vi "PerformCalibrationMultiMixture.vi"(0 "MFCS_EZ":T3, 1 "Total Flow Setpoint":dbl, 2 "Ctr Water Valve":u16(ring) items=["A1", "A2", "A3", "A4", "B1", "B2", "B3", "B4", "B5", "B6", "B7", "B8", "A5", "A6", "A7", "A8"], 3 "Calibration Mode":T2(ring), 5 "Calibration Refs":T1, 7 "Manual Default Set Pressures":dbl[](array[numeric]), 12 "Total Odor Flow":dbl, 13 "Water Mix Valve":u16(ring) items=["A1", "A2", "A3", "A4", "B1", "B2", "B3", "B4", "B5", "B6", "B7", "B8", "A5", "A6", "A7", "A8", ""]) -> (4 "Ctr Pressure":dbl, 6 "Set Pressures Out":dbl[](array[numeric]), 10 "New Manual Pressure":dbl[](array[numeric]), 15 "Aborted?":bool)   [LabVIEW 2016]
uses:
  <userlib>/Fluigent/Fluigent MFCS/FluigentMFCS_Full.llb/_EZmfcsRefNum.ctl
  <userlib>/Fluigent/Fluigent MFCS/FluigentMFCS_Full.llb/_EZmfcsEnum.ctl
  <userlib>/Fluigent/Fluigent MFCS/FluigentMFCS_Full.llb/MFCS_EZ Write Channel Pressure.vi
  <userlib>/Fluigent/Fluigent MFCS/FluigentMFCS_Full.llb/MFCS_EZ Read All Channels Pressure.vi
  <vilib>/Utility/miscctls.llb/LVStringsAndValuesArrayTypeDef.ctl
panel:
  out "odor starting pressure":dbl
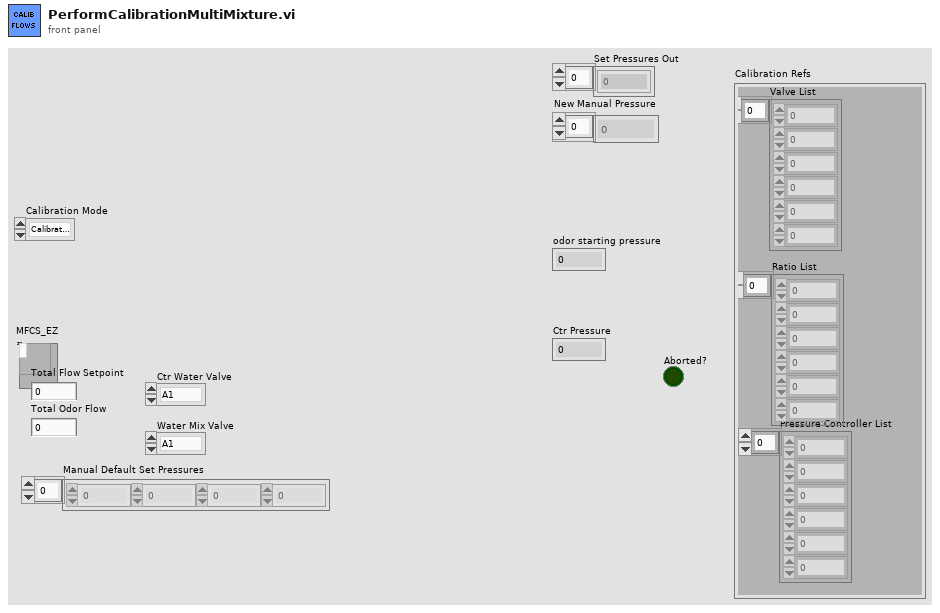
[diagram p1: front panel]
types:
  T1 = cluster{"Pressure Controller List":u8[], "Ratio List":dbl[], "Valve List":u16[]}
  T2 = enum16{"Calibrate All", "Control Only", "Odors Only"}
  T3 = typedef "_EZmfcsRefNum.ctl" = refnum<k1>
  T4 = cluster{enum16{"A", "B", "C"}[], enum16{"1", "2", "3", "4", "5", "6", "7", "8"}[], bool[]}[]
  T5 = typedef "LVStringsAndValuesArrayTypeDef.ctl" = cluster{"String":string, "Value":ext}[]
  T6 = enum16{"Release", "Create", "Send", "Wait", "Cancel"}
  T7 = cluster{enum16{"A", "B", "C"}[], enum16{"1", "2", "3", "4", "5", "6", "7", "8"}[], bool[]}
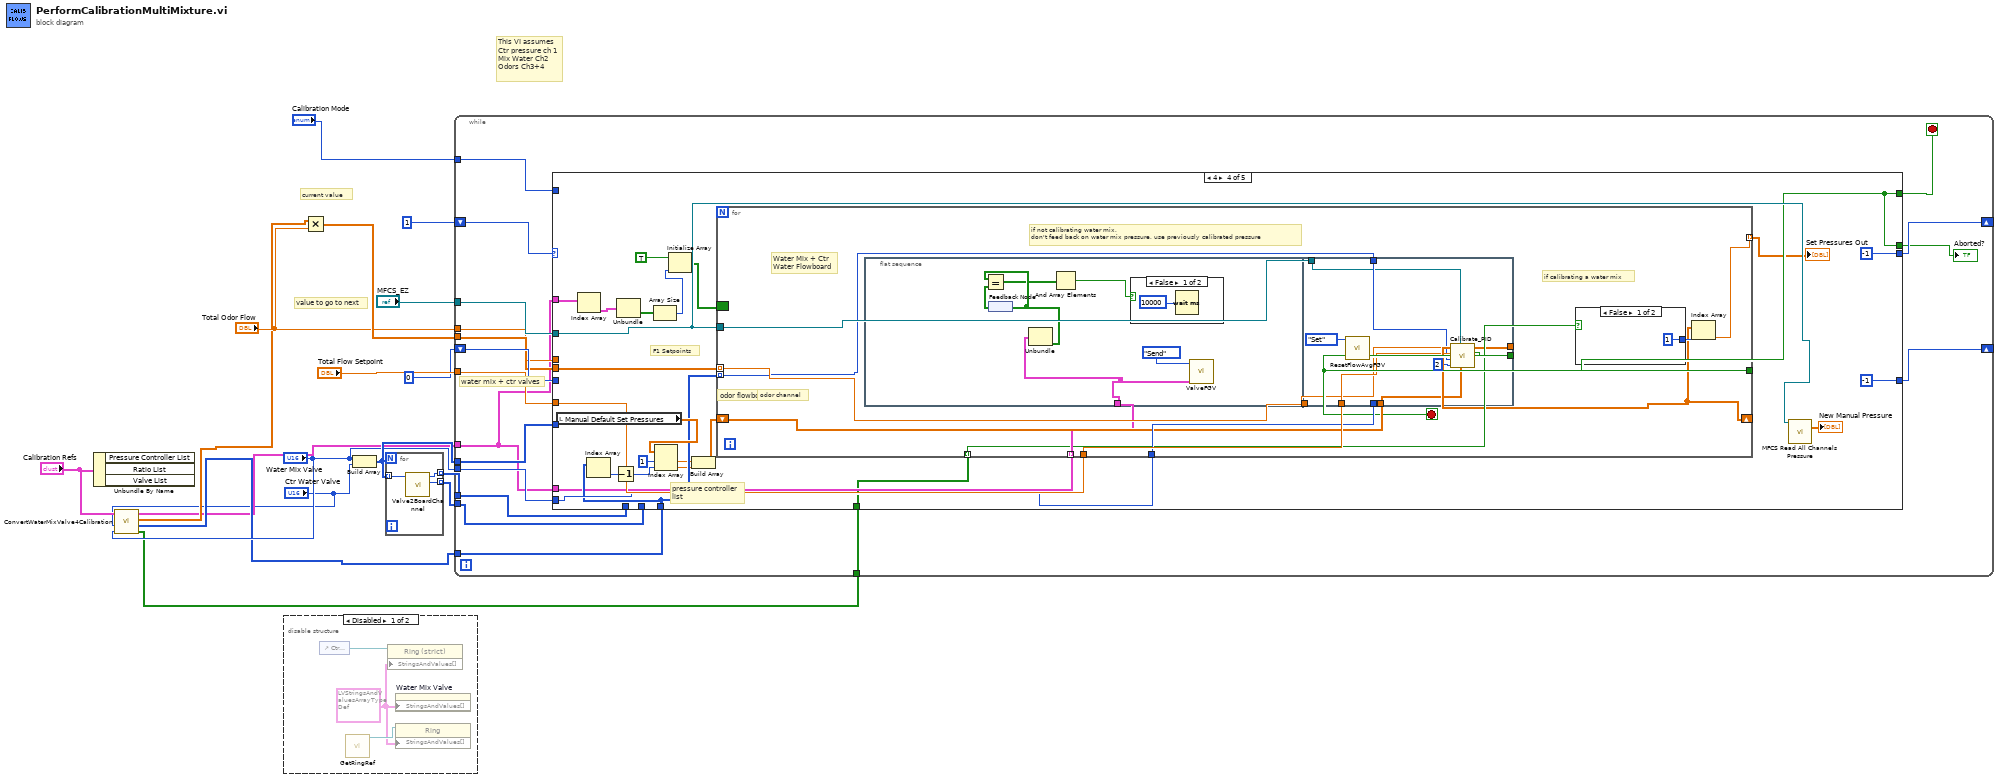
[diagram p0: block diagram]
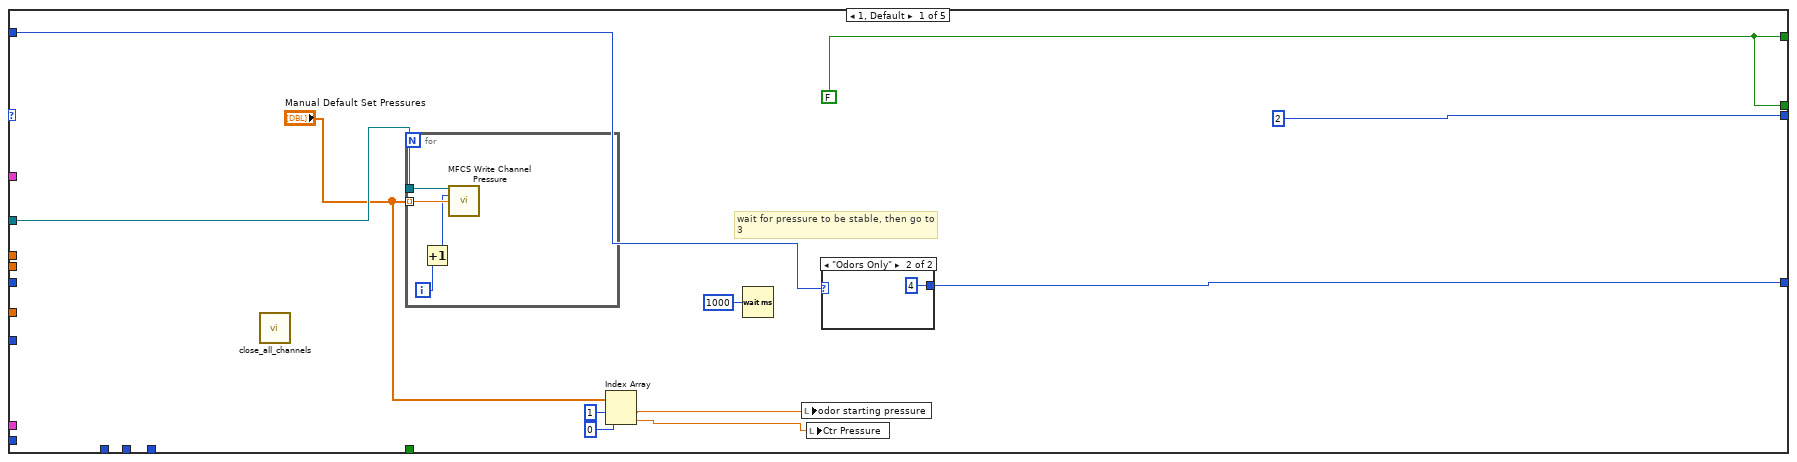
[diagram p3: hidden frame]
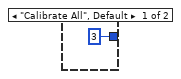
[diagram p4: hidden frame]
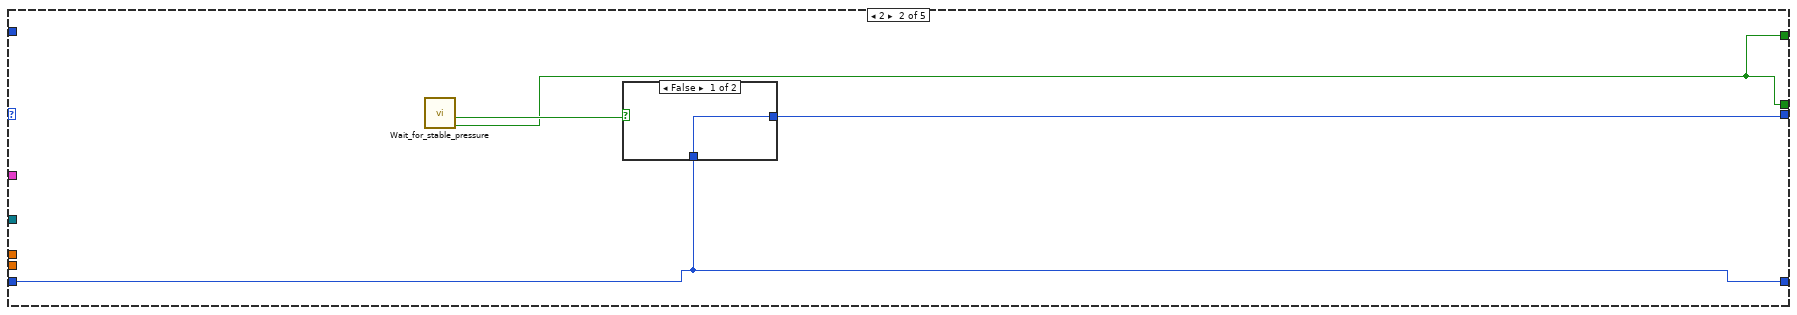
[diagram p5: hidden frame]
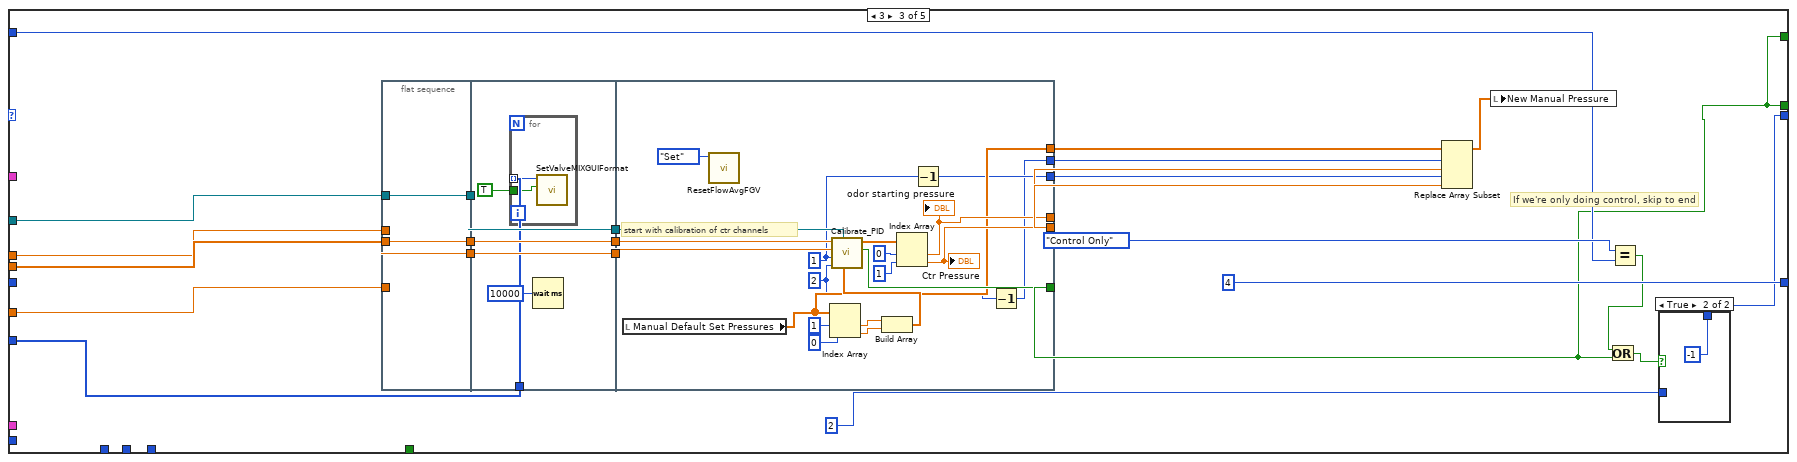
[diagram p7: hidden frame]
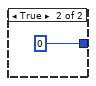
[diagram p9: hidden frame]
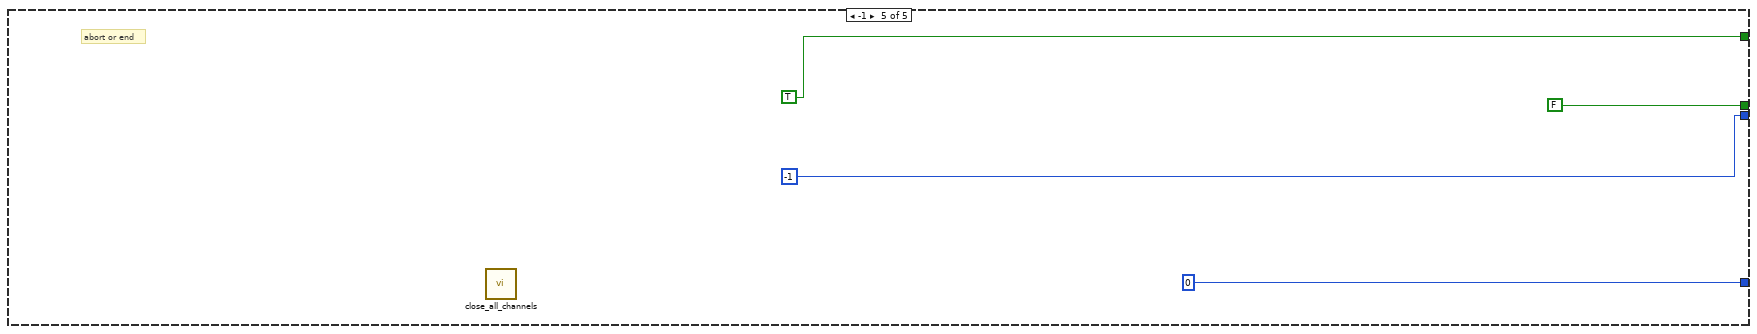
[diagram p11: hidden frame]
diagram:
  # "This VI assumes \nCtr pressure ch 1\nMix Water Ch2\nOdors Ch3+4"
  # "current value"
  # "value to go to next"
  n1 = Unbundle By Name("Calibration Refs") -> ()  [unwired: 3 out]
  n2 = call "ConvertWaterMixValve4Calibration.vi"("Water Mix Valve"="Water Mix Valve", "Ctr Water Valve"="Ctr Water Valve", "Calibration Refs"="Calibration Refs") -> ("Water Calibration?"=w2:bool[], "PressList"=w5:u8[], "RatioList"=w4:dbl[], "Valve Signal Array"=w3:T4)  [unwired: 5 in]
  n3 = disable-structure shown="Disabled" {
    frame Disabled {
      w18 = T5 [{"String"="A1", "Value"=0.0}, {"String"="A2", "Value"=1.0}, {"String"="A3", "Value"=2.0}, {"String"="A4", "Value"=3.0}, {"String"="B1", "Value"=4.0}, {"String"="B2", "Value"=5.0}, {"String"="B3", "Value"=6.0}, {"String"="B4", "Value"=7.0}, {"String"="B5", "Value"=8.0}, {"String"="B6", "Value"=9.0}, {"String"="B7", "Value"=10.0}, {"String"="B8", "Value"=11.0}, {"String"="A5", "Value"=12.0}] ("Master Valves")
      n4 = control-ref of="Ctr Water Valve"() -> (w19:refnum<vi>)
      n5 = call "GetRingRef.vi"() -> ("Ring Reference"=w20:refnum<vi>, "Array Reference"=w21:refnum<vi>)  [unwired: 9 in, 1 out]
      n6 = property on="Property Node" class="Ring (strict)"(reference=w19, "StringsAndValues[]"=w18) -> ()  [unwired: 1 in, 2 out]
      n7 = property on="Water Mix Valve" class="Ring (strict)"("StringsAndValues[]"=w18) -> ()  [unwired: 2 in, 2 out]
      n8 = property class="Ring"(reference=w20, "StringsAndValues[]"=w18) -> ()  [unwired: 1 in, 2 out]
    }
    frame Enabled {
    }
  }
  n9 = Multiply(x=w4, y="Total Odor Flow") -> (x*y=w10:dbl[])
  n10 = Build Array("Water Mix Valve", "Ctr Water Valve") -> (w13:u16[])
  n11 = for {
    tunnel: w13 -> [w24] mode=indexing
    tunnel: [w23] -> w12 mode=indexing
    tunnel: [w22] -> w11 mode=indexing
    n12 = call "Valve2BoardChannel.vi"("ValveID"=w24) -> ("Channel"=w22:enum16{"1", "2", "3", "4", "5", "6", "7", "8"}, "Flowboard"=w23:enum16{"A", "B", "C"})  [unwired: 9 in]
  }
  n13 = while {
    tunnel: "MFCS_EZ" -> [w42]
    tunnel: "Total Flow Setpoint" -> [w41]
    shift-right: [w39] -> _
    shift-left: 1 -> [w40]
    tunnel: w13 -> [w38]
    shift-right: [w37] -> _
    shift-left: 0 -> [w36]
    tunnel: w5 -> [w29]
    tunnel: w12 -> [w35]
    tunnel: w11 -> [w34]
    tunnel: w10 -> [w33]
    tunnel: "Water Mix Valve" -> [w31]
    tunnel: "Total Odor Flow" -> [w32]
    tunnel: "Calibration Mode" -> [w30]
    tunnel: w3 -> [w25]
    tunnel: w2 -> [w28]
    stop <- w27 stop-if-true
    # "pressure controller \nlist"
    # "water mix + ctr valves"
    n14 = case shown="4" w40 {
      tunnel: w42 -> [w52 _ w90 w133 _]
      tunnel: w33 -> [_ _ w89 w147 _]
      tunnel: w41 -> [_ _ w88 w148 _]
      tunnel: [w43 w60 w66 w131 TRUE] -> w27
      tunnel: [2 w63 w78 -1 -1] -> w39
      tunnel: w38 -> [_ _ w73 _ _]
      tunnel: [w51 w62 4 -1 0] -> w37
      tunnel: w36 -> [_ w62 _ _ _]
      tunnel: w29 -> [_ _ _ w140 _]
      tunnel: w35 -> [_ _ _ _ _]
      tunnel: w34 -> [_ _ _ _ _]
      tunnel: w31 -> [_ _ _ w146 _]
      tunnel: w32 -> [_ _ w81 _ _]
      tunnel: w30 -> [w49 _ w75 _ _]
      tunnel: w25 -> [_ _ _ w135 _]
      tunnel: w28 -> [_ _ _ w134 _]
      tunnel: [w43 w60 w66 w131 FALSE ("Aborted?")] -> w26
      tunnel: w25 -> [_ _ _ w129 _]
      frame 1, Default {
        w43 = FALSE
        # "wait for pressure to be stable, then go to\n3"
        n15 = call "close_all_channels.vi"() -> ()  [unwired: 12 in]
        n16 = for {
          tunnel: "Manual Default Set Pressures" -> [w59] mode=indexing
          tunnel: w52 -> [w57]
          i -> [w58]
          n17 = Increment(x=w58) -> (x+1=w56:i32)
          n18 = call-poly <userlib>:"MFCS Write Channel Pressure.vi"("MFCS_EZ"=w57, "Channel Number (default=1)"=w56, "Pressure (mBar)"=w59) -> ()  [unwired: 11 in, 2 out]
        }
        n19 = Index Array(array="Manual Default Set Pressures", index #1=1 ("index"), index #2=0 ("index")) -> (element #1=w46:dbl, element #2=w45:dbl)
        n20 = Wait (ms)(milliseconds to wait=u32 1000) -> ()  [unwired: 1 out]
        n21 = local write "odor starting pressure"(w46) -> ()
        n22 = local write "Ctr Pressure"(w45) -> ()
        n23 = case shown="\"Odors Only\"" w49 {
          tunnel: [3 4] -> w51
          frame "Calibrate All", Default {
          }
          frame "Odors Only" {
          }
        }
      }
      frame 2 {
        n24 = call "Wait_for_stable_pressure.vi"() -> ("Aborted?"=w60:bool, "Pressure Stable?"=w61:bool)  [unwired: 8 in]
        n25 = case shown="False" w61 {
          tunnel: [w64 w65] -> w63
          tunnel: w62 -> [w64 w65]
          frame False {
          }
          frame True {
          }
        }
      }
      frame 3 {
        # "If we're only doing control, skip to end"
        n26 = flat-sequence {
          tunnel: w88 -> [w94]
          tunnel: w89 -> [_]
          tunnel: w90 -> [w95]
          tunnel: [w95] -> w87
          tunnel: [w94] -> w84
          tunnel: w81 -> [w93]
          tunnel: [w93] -> w80
          tunnel: w87 -> [w101]
          tunnel: [w101] -> w86
          tunnel: [w100] -> w85
          tunnel: w84 -> [w99]
          tunnel: [w99] -> w83
          tunnel: w73 -> [w97]
          tunnel: w80 -> [w100]
          tunnel: w86 -> [w123]
          tunnel: w85 -> [w122]
          tunnel: w83 -> [w121]
          tunnel: [w114] -> w66
          tunnel: [w104] -> w72
          tunnel: [w105] -> w71
          tunnel: [w110] -> w70
          tunnel: [w109] -> w69
          tunnel: [w108] -> w67
          frame #0 {
          }
          frame #1 {
            n27 = for {
              tunnel: TRUE ("State") -> [w103]
              tunnel: w97 -> [w102] mode=indexing
              n28 = call "SetValveMIXGUIFormat.vi"("State"=w103, "ValveID"=w102) -> ()  [unwired: 10 in]
            }
            n29 = Wait (ms)(milliseconds to wait=u32 10000) -> ()  [unwired: 1 out]
          }
          frame #2 {
            w106 = i16 1 ("Odor Mix Pressure Channel")
            w107 = i16 2 ("Water Mix Pressure Channel")
            # "start with calibration of ctr channels"
            n30 = local read "Manual Default Set Pressures"() -> (w108:dbl[])
            n31 = call "ResetFlowAvgFGV.vi"("Action"=enum16{"Create", "Set", "Wait"}."Set") -> ()  [unwired: 10 in, 1 out]
            n32 = Index Array(array=w108, index #1=1 ("index"), index #2=0 ("index")) -> (element #1=w116:dbl, element #2=w117:dbl)
            n33 = Build Array(w116, w117) -> (w115:dbl[])
            n34 = call "Calibrate_PID.vi"("Starting Pressure"=w115, "MFCS_EZ"=w123, "Water Mix Pressure Channel"=w107, "Odor Mix Pressure Channel"=w106, "Ftot Setpoint"=w121, "F1 Setpoint"=w122) -> ("Aborted?"=w114:bool, "Set Pressure Out"=w120:dbl[])  [unwired: 4 in]
            n35 = Index Array(array=w120, index #1=0 ("index"), index #2=1 ("index")) -> (element #1=w109:dbl, element #2=w110:dbl)
            "Ctr Pressure" <- w110
            "odor starting pressure" <- w109
            n36 = Decrement(x=w106) -> (x-1=w105:i16)
            n37 = Decrement(x=w107) -> (x-1=w104:i16)
          }
        }
        n38 = Replace Array Subset(array=w67, new element #1=w69, index #1=w72, new element #2=w70, index #2=w71) -> (w68:dbl[])
        n39 = local write "New Manual Pressure"(w68) -> ()
        n40 = Equal?(x=T2."Control Only" ("Calibration Mode"), y=w75) -> (x = y?=w74:bool)
        n41 = Or(x=w74, y=w66) -> (x .or. y?=w77:bool)
        n42 = case shown="True" w77 {
          tunnel: 2 -> [w91 _]
          tunnel: [w91 -1] -> w78
          frame False {
          }
          frame True {
          }
        }
      }
      frame 4 {
        # "F1 Setpoints"
        n43 = local read "Manual Default Set Pressures"() -> (w142:dbl[])
        n44 = Index Array(array=w129) -> (element=w128:T7)  [unwired: 1 in]
        n45 = Index Array(array=w140) -> (element=w139:u8)  [unwired: 1 in]
        n46 = Decrement(x=w139) -> (x-1=w138:u8)
        n47 = Unbundle(w128) -> (w127:bool[])  [unwired: 2 out]
        n48 = Array Size(array=w127) -> (size(s)=w126:i32)
        n49 = Index Array(array=w142, index #1=1 ("index"), index #2=w138) -> (element #1=w136:dbl, element #2=w137:dbl)
        n50 = Initialize Array(TRUE, w126) -> (w124:bool[])
        n51 = Build Array(w136, w137) -> (w143:dbl[])
        n52 = for {
          tunnel: w140 -> [w154] mode=indexing
          tunnel: w148 -> [w160]
          tunnel: w133 -> [w159]
          tunnel: w147 -> [w158] mode=indexing
          tunnel: w146 -> [w157]
          shift-right: [w150] -> _
          shift-left: w143 -> [w156]
          tunnel: [w155] -> w131
          tunnel: w135 -> [w153] mode=indexing
          tunnel: w134 -> [w152] mode=indexing
          tunnel: [w149] -> w130 mode=indexing
          border: w124 -> [_]
          stop <- w155 stop-if-true
          # "if not calibrating water mix, \ndon't feed back on water mix pressure, use previously calibrated pressure"
          # "if calibrating a water mix"
          # "odor channel"
          # "odor flowboard"
          # "Water Mix + Ctr \nWater Flowboard"
          n53 = flat-sequence {
            tunnel: w153 -> [w167]
            tunnel: w160 -> [w178]
            tunnel: w159 -> [w170]
            tunnel: w158 -> [w177]
            tunnel: [w176] -> w155
            tunnel: [w175] -> w150
            tunnel: w154 -> [w174]
            tunnel: w157 -> [_]
            tunnel: w156 -> [w172]
            frame #0 {
              n54 = feedback #1() -> (w166:bool[])
              n55 = Unbundle(w167) -> (w165:bool[])  [unwired: 2 out]
              n56 = Equal?(x=w165, y=w166) -> (x = y?=w164:bool[])
              n57 = feedback-in #1(w165) -> ()
              n58 = And Array Elements(Boolean array=w164) -> (logical AND=w163:bool)
              n59 = case shown="False" w163 {
                frame False {
                  n60 = Wait (ms)(milliseconds to wait=u32 10000) -> ()  [unwired: 1 out]
                }
                frame True {
                }
              }
              n61 = call "ValveFGV.vi"("Valve Data"=w167, "Action"=T6."Send") -> ()  [unwired: 6 in, 4 out]
            }
            frame #1 {
              n62 = call "ResetFlowAvgFGV.vi"("Action"=enum16{"Create", "Set", "Wait"}."Set") -> ()  [unwired: 10 in, 1 out]
              n63 = call "Calibrate_PID.vi"("Starting Pressure"=w172, "MFCS_EZ"=w170, "Water Mix Pressure Channel"=i16 2, "Odor Mix Pressure Channel"=w174, "Ftot Setpoint"=w178, "F1 Setpoint"=w177) -> ("Aborted?"=w176:bool, "Set Pressure Out"=w175:dbl[])  [unwired: 4 in]
            }
          }
          n64 = case shown="False" w152 {
            tunnel: [1 0] -> w151
            frame False {
            }
            frame True {
            }
          }
          n65 = Index Array(array=w150, index=w151) -> (element=w149:dbl)
        }
        "Set Pressures Out" <- w130
        n66 = call-poly <userlib>:"MFCS Read All Channels Pressure.vi"("MFCS_EZ"=w133) -> ("All Channels Pressure"=→"New Manual Pressure":dbl[])  [unwired: 12 in, 2 out]
      }
      frame -1 {
        # "abort or end"
        n67 = call "close_all_channels.vi"() -> ()  [unwired: 12 in]
      }
    }
    "Aborted?" <- w26
  }
